vi "Motion@Config__Parameter.vi"(1 "ParamterIn":string) -> (0 "ParamterOut":string)   [LabVIEW 2019]
panel:
  in  "Axis":string(combo)="Scale"
  in  "Value":string(combo)
  in  "Parameter":string(combo)="Scale"
  in  "MotorName":string(combo)
  in  "Confirm":bool
  # "Motor@Config $Motor,$Axis,$Parameter,$Value"
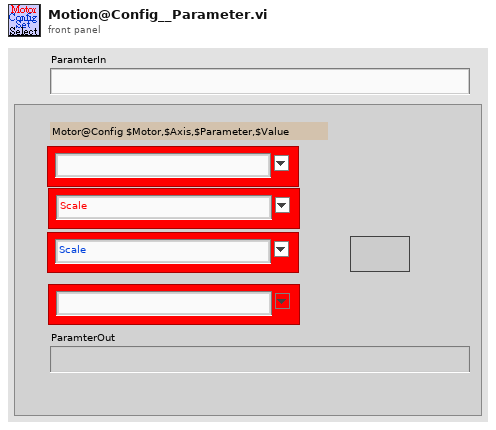
[diagram p1: front panel]
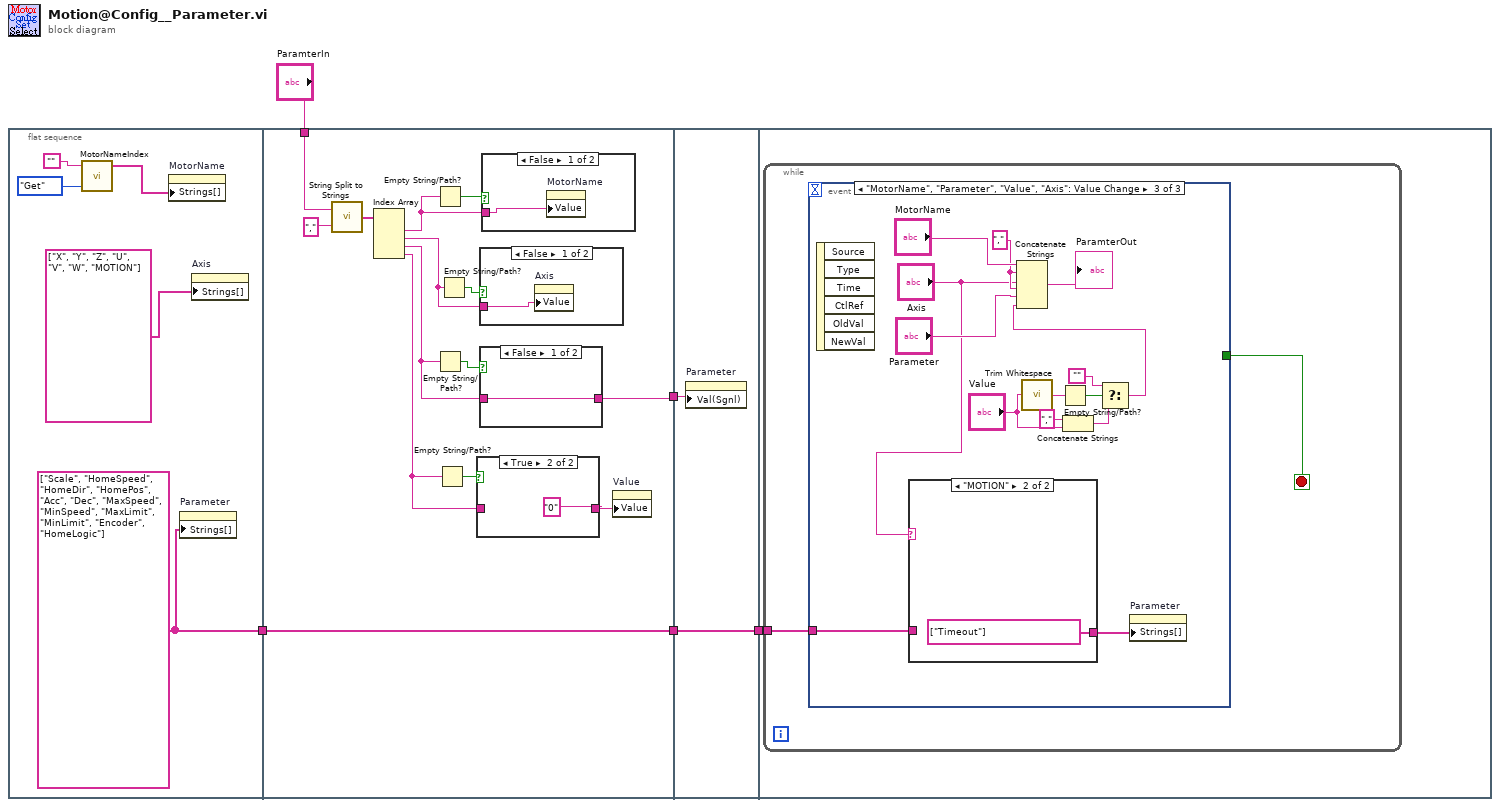
[diagram p0: block diagram]
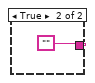
[diagram p4: hidden frame]
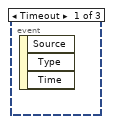
[diagram p6: hidden frame]
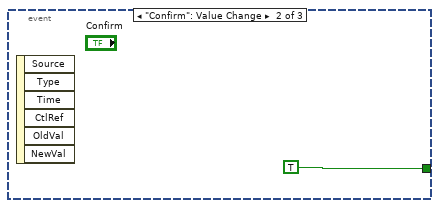
[diagram p7: hidden frame]
diagram:
  n1 = flat-sequence {
    tunnel: [w6] -> w1
    tunnel: "ParamterIn" -> [w22]
    tunnel: [w16] -> w4
    tunnel: [w11] -> w2
    tunnel: w1 -> [w11]
    tunnel: w4 -> [w32]
    tunnel: [w31] -> w3
    tunnel: w2 -> [w31]
    tunnel: w3 -> [w33]
    frame #0 {
      w6 = string[] ["Scale", "HomeSpeed", "HomeDir", "HomePos", "Acc", "Dec", "MaxSpeed", "MinSpeed", "MaxLimit", "MinLimit", "Encoder", "HomeLogic"]
      n2 = call "MotorNameIndex.vi"("OP"=enum16{"Get", "Update", "Init"}."Get", "MotorName"="") -> ("MotorList"=w8:string[])  [unwired: 1 in, 2 out]
      n3 = property on="MotorName" class="CmbBox"("Strings[]"=w8) -> ()  [unwired: 2 in, 2 out]
      n4 = property on="Parameter" class="CmbBox"("Strings[]"=w6) -> ()  [unwired: 2 in, 2 out]
      n5 = property on="Axis" class="CmbBox"("Strings[]"=string[] ["X", "Y", "Z", "U", "V", "W", "MOTION"] ("Strings []")) -> ()  [unwired: 2 in, 2 out]
    }
    frame #1 {
      n6 = call "String Split to Strings.vi"("search string/char (-)"=",", "String"=w22) -> ("Array"=w24:string[])
      n7 = Index Array(array=w24) -> (element #1=w20:string, element #2=w12:string, element #3=w14:string, element #4=w15:string)  [unwired: 4 in]
      n8 = Empty String/Path?(string/path=w20) -> (empty?=w21:bool)
      n9 = Empty String/Path?(string/path=w14) -> (empty?=w19:bool)
      n10 = Empty String/Path?(string/path=w15) -> (empty?=w18:bool)
      n11 = Empty String/Path?(string/path=w12) -> (empty?=w13:bool)
      n12 = case shown="True" w18 {
        tunnel: [w26 "0"] -> w17
        tunnel: w15 -> [w26 _]
        frame False {
        }
        frame True {
        }
      }
      n13 = case shown="False" w13 {
        tunnel: w12 -> [w25 _]
        frame False {
          n14 = property on="Axis" class="CmbBox"("Value"=w25) -> ()  [unwired: 2 in, 2 out]
        }
        frame True {
        }
      }
      n15 = case shown="False" w19 {
        tunnel: [w28 ""] -> w16
        tunnel: w14 -> [w28 _]
        frame False {
        }
        frame True {
        }
      }
      n16 = case shown="False" w21 {
        tunnel: w20 -> [w30 _]
        frame False {
          n17 = property on="MotorName" class="CmbBox"("Value"=w30) -> ()  [unwired: 2 in, 2 out]
        }
        frame True {
        }
      }
      n18 = property on="Value" class="CmbBox"("Value"=w17) -> ()  [unwired: 2 in, 2 out]
    }
    frame #2 {
      n19 = property on="Parameter" class="CmbBox"("Val(Sgnl)"=w32) -> ()  [unwired: 2 in, 2 out]
    }
    frame #3 {
      n20 = while {
        tunnel: w33 -> [w34]
        stop <- w35 stop-if-true
        n21 = event shown="[2] \"MotorName\", \"Parameter\", \"Value\", \"Axis\": Value Change" {
          selector: _ -> [_ _ _]
          dyn-events: _ -> [_ _ _]
          timeout: _ -> [_ _ _]
          tunnel: [_ TRUE _] -> w35
          tunnel: w34 -> [_ _ w38]
          event Timeout {
            n22 = event-data() -> ()  [unwired: 1 in, 3 out]
          }
          event "Confirm": Value Change {
            n23 = event-data() -> ()  [unwired: 1 in, 6 out]
          }
          event "MotorName", "Parameter", "Value", "Axis": Value Change {
            w42 = "," ("string")
            n24 = event-data() -> ()  [unwired: 1 in, 6 out]
            n25 = case shown="\"MOTION\"" "Axis" {
              tunnel: w38 -> [w51 _]
              tunnel: [w51 string[] ["Timeout"]] -> w37
              frame "False", Default {
              }
              frame "MOTION" {
              }
            }
            n26 = call <vilib>:"Trim Whitespace.vi"("string"="Value") -> ("trimmed string"=w44:string)  [unwired: 1 in]
            n27 = Empty String/Path?(string/path=w44) -> (empty?=w45:bool)
            n28 = Concatenate Strings("," ("string"), "Value") -> (w47:string)
            n29 = Select(t="", s=w45, f=w47) -> (s? t:f=w41:string)
            n30 = Concatenate Strings("MotorName", w42, "Axis", w42, "Parameter", w41) -> (→"ParamterOut":string)
            n31 = property on="Parameter" class="CmbBox"("Strings[]"=w37) -> ()  [unwired: 2 in, 2 out]
          }
        }
      }
    }
  }
